vi "LightPresetButtons.vi"(10 "Lights Values":T1=[[{"Port"=1, "On Value"=255, "Off Value"=255}, {"Port"=2, "On Value"=0, "Off Value"=0}, {"Port"=3, "On Value"=0, "Off Value"=0}], [{"Port"=4, "On Value"=0, "Off Value"=0}, {"Port"=5, "On Value"=0, "Off Value"=0}, {"Port"=6, "On Value"=0, "Off Value"=0}], [{"Port"=7, "On Value"=0, "Off Value"=0}, {"Port"=8, "On Value"=0, "Off Value"=0}, {"Port"=9, "On Value"=0, "Off Value"=0}], [{"Port"=10, "On Value"=0, "Off Value"=0}, {"Port"=11, "On Value"=0, "Off Value"=0}, {"Port"=12, "On Value"=0, "Off Value"=0}], [{"Port"=13, "On Value"=0, "Off Value"=0}, {"Port"=14, "On Value"=0, "Off Value"=0}, {"Port"=15, "On Value"=0, "Off Value"=0}], [{"Port"=58, "On Value"=255, "Off Value"=0}, {"Port"=0, "On Value"=0, "Off Value"=0}, {"Port"=0, "On Value"=0, "Off Value"=0}], [{"Port"=49, "On Value"=255, "Off Value"=0}, {"Port"=0, "On Value"=0, "Off Value"=0}, {"Port"=0, "On Value"=0, "Off Value"=0}], [{"Port"=52, "On Value"=255, "Off Value"=0}, {"Port"=0, "On Value"=0, "Off Value"=0}, {"Port"=0, "On Value"=0, "Off Value"=0}], [{"Port"=55, "On Value"=255, "Off Value"=0}, {"Port"=0, "On Value"=0, "Off Value"=0}, {"Port"=0, "On Value"=0, "Off Value"=0}], [{"Port"=46, "On Value"=255, "Off Value"=0}, {"Port"=0, "On Value"=0, "Off Value"=0}, {"Port"=0, "On Value"=0, "Off Value"=0}], [{"Port"=61, "On Value"=0, "Off Value"=0}, {"Port"=0, "On Value"=0, "Off Value"=0}, {"Port"=0, "On Value"=0, "Off Value"=0}]], 11 "output cluster":T2) -> (1 "MaxnbTotesUnder":i32, 2 "CurrentPosition":dbl)   [LabVIEW 2014]
uses:
  <vilib>/Rock Robotics/Network Tables/SD Read Number.vi
  PresetValues.ctl
  LEDdriver/LEDPorts.ctl
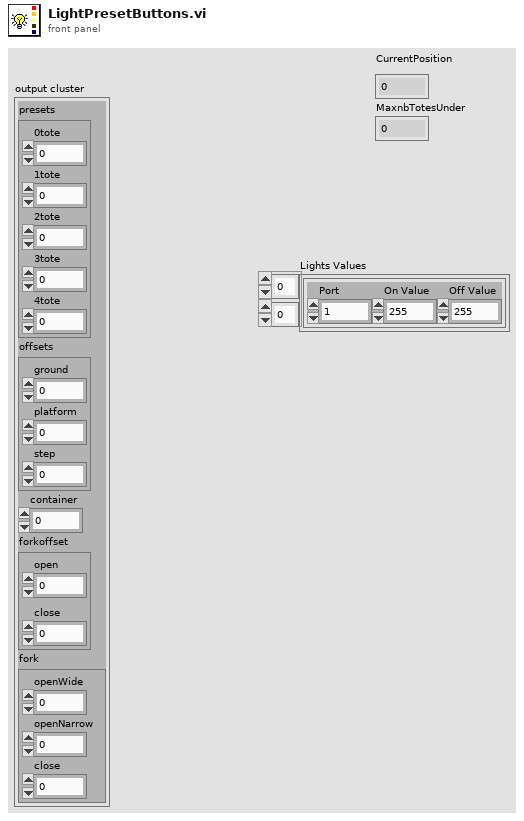
[diagram p1: front panel]
types:
  T1 = typedef "LEDPorts.ctl" = cluster{"Port":i16, "On Value":u8, "Off Value":u8}[][]
  T2 = typedef "PresetValues.ctl" = cluster{"presets":cluster{"0tote":dbl, "1tote":dbl, "2tote":dbl, "3tote":dbl, "4tote":dbl}, "offsets":cluster{"ground":dbl, "platform":dbl, "step":dbl}, "container":dbl, "forkoffset":cluster{"open":dbl, "close":dbl}, "fork":cluster{"openWide":dbl, "openNarrow":dbl, "close":dbl}}
  T3 = cluster{"0tote":dbl, "1tote":dbl, "2tote":dbl, "3tote":dbl, "4tote":dbl}
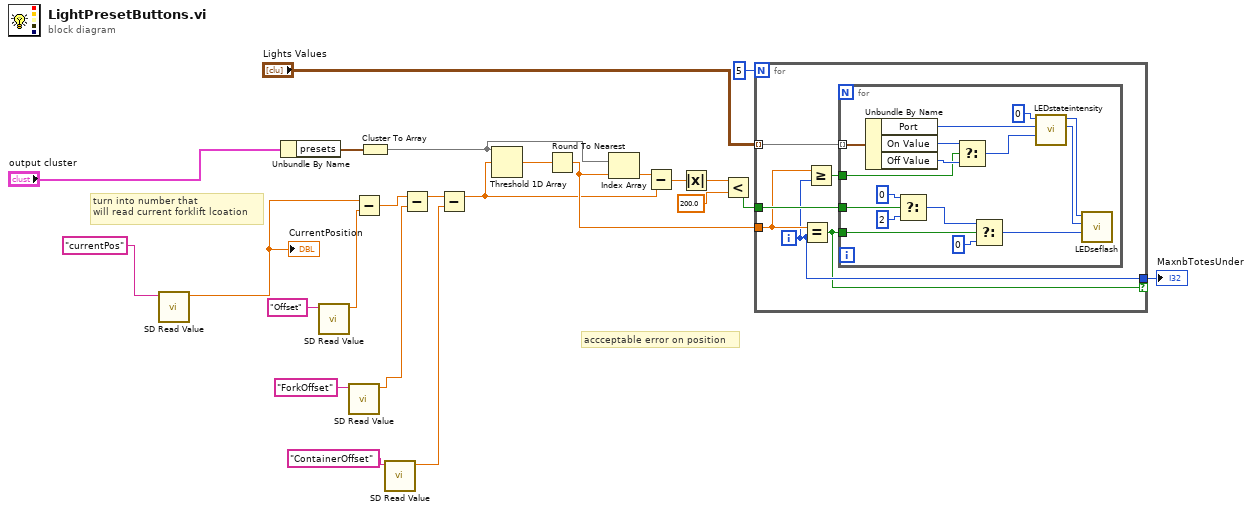
[diagram p0: block diagram]
diagram:
  # "accceptable error on position"
  # "turn into number that\nwill read current forklift lcoation"
  n1 = call-poly <vilib>:"SD Read Value.vi"("Name"="currentPos") -> ("Numeric"=w15:dbl)  [unwired: 8 in, 2 out]
  "CurrentPosition" <- w15
  n2 = Unbundle By Name("output cluster") -> ("presets"=w24:T3)
  n3 = call-poly <vilib>:"SD Read Value.vi"("Name"="Offset") -> ("Numeric"=w14:dbl)  [unwired: 8 in, 2 out]
  n4 = call-poly <vilib>:"SD Read Value.vi"("Name"="ForkOffset") -> ("Numeric"=w4:dbl)  [unwired: 8 in, 2 out]
  n5 = Subtract(x=w15, y=w14) -> (x-y=w18:dbl)
  n6 = Cluster To Array(cluster=w24) -> (array=w22:dbl[])
  n7 = call-poly <vilib>:"SD Read Value.vi"("Name"="ContainerOffset") -> ("Numeric"=w2:dbl)  [unwired: 8 in, 2 out]
  n8 = Subtract(x=w18, y=w4) -> (x-y=w5:dbl)
  n9 = Subtract(x=w5, y=w2) -> (x-y=w3:dbl)
  n10 = Threshold 1D Array(2:w3, 3:w22) -> (0:w16:dbl)  [unwired: 1 in]
  n11 = Round To Nearest(number=w16) -> (nearest integer value=w9:dbl)
  n12 = Index Array(array=w22, index=w9) -> (element=w17:dbl)
  n13 = Subtract(x=w17, y=w3) -> (x-y=w19:dbl)
  n14 = Absolute Value(x=w19) -> (abs(x)=w20:dbl)
  n15 = Less?(x=w20, y=200.0) -> (x < y?=w8:bool)
  n16 = for {
    N: 5 -> [_]
    tunnel: "Lights Values" -> [w30] mode=indexing
    tunnel: w9 -> [w28]
    tunnel: w8 -> [w29]
    tunnel: [w26] -> w1 if=w25
    i -> [w26]
    n17 = Equal?(x=w28, y=w26) -> (x = y?=w25:bool)
    n18 = Greater Or Equal?(x=w28, y=w26) -> (x >= y?=w27:bool)
    n19 = for {
      tunnel: w30 -> [w43] mode=indexing
      tunnel: w25 -> [w38]
      tunnel: w29 -> [w34]
      tunnel: w27 -> [w31]
      n20 = Unbundle By Name(w43) -> ("Port"=w42:i16, "On Value"=w41:u8, "Off Value"=w40:u8)
      n21 = Select(t=u8 0, s=w34, f=u8 2) -> (s? t:f=w35:u8)
      n22 = Select(t=w41, s=w31, f=w40) -> (s? t:f=w39:u8)
      n23 = Select(t=w35, s=w38, f=u8 0) -> (s? t:f=w36:u8)
      n24 = call "LEDstateintensity.vi"("intensity"=w39, "port"=w42, "Id"=i16 0) -> ("port out"=w44:i16, "Id out"=w45:i16)  [unwired: 6 in, 1 out]
      n25 = call "LEDseflash.vi"("flashspeed"=w36, "port"=w44, "Id"=w45) -> ()  [unwired: 8 in, 1 out]
    }
  }
  "MaxnbTotesUnder" <- w1
